vi "Prepend to Log.vi"(10 "new entry":string) -> (11 "Log out":string)   [LabVIEW 2023, in "Message Queue Helper.lvlib"]
uses:
  Message Queue Helper.lvlib
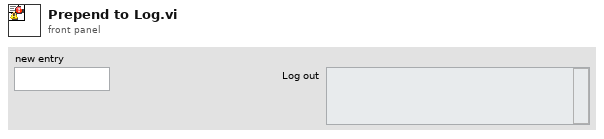
[diagram p1: front panel]
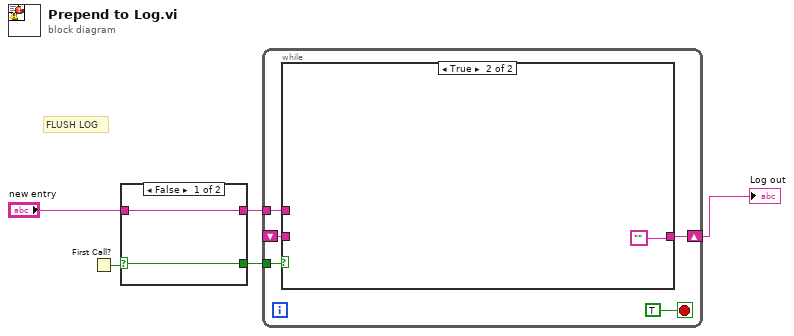
[diagram p0: block diagram]
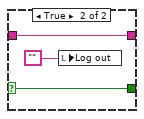
[diagram p2: hidden frame]
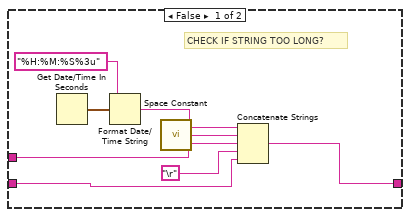
[diagram p3: hidden frame]
diagram:
  # "FLUSH LOG"
  n1 = First Call?() -> (First Call?: T/F=w2:bool)
  n2 = case shown="False" w2 {
    selector: w2 -> [w6 w8]
    tunnel: "new entry" -> [w7 w10]
    tunnel: [w7 w10] -> w3
    tunnel: [w6 w8] -> w1
    frame False {
    }
    frame True {
      n3 = local write "Log out"("") -> ()
    }
  }
  n4 = while {
    tunnel: w3 -> [w14]
    shift-right: [w13] -> w5
    shift-left: _ -> [w12]
    tunnel: w1 -> [w11]
    stop <- TRUE stop-if-true
    n5 = case shown="True" w11 {
      tunnel: w14 -> [w18 _]
      tunnel: [w17 ""] -> w13
      tunnel: w12 -> [w16 _]
      frame False {
        # "CHECK IF STRING TOO LONG?"
        n6 = Get Date/Time In Seconds() -> (seconds since 1Jan1904=w23:timestamp)
        n7 = Format Date/Time String(time format string (%c)="%H:%M:%S%3u", seconds (now)=w23) -> (date/time string=w20:string)  [unwired: 1 in]
        n8 = call <vilib>:"Space Constant.vi"() -> ("String"=w21:string)
        n9 = Concatenate Strings(w20, w21, w18, "\r", w16) -> (w17:string)
      }
      frame True {
      }
    }
  }
  "Log out" <- w5
